vi "LVClass_WavefrontCorrector Check User Preferences.vi"(0 "WavefrontCorrector in":refnum<class "WavefrontCorrector.lvclass">, 5 "Mirror preferences":T1, 11 "error in (no error)":errorcluster) -> (4 "WavefrontCorrector out":refnum<class "WavefrontCorrector.lvclass">, 15 "error out":errorcluster)   [LabVIEW 2020, in "WavefrontCorrector.lvclass"]
doc: "Assert requested preferences fulfill specifications constraints.\n\n--------------------------------------------------------------------------------\n\n<B>correctorIn </B> : WavefrontCorrector object.\n<B>correctorOut </B> : WavefrontCorrector object.\n<B>sleep_after_movement </B> : WavefrontCorrector preferences : Time to stabilization (ms).\n<B>min </B> : WavefrontCorrector preferences : lowest command value.\n<B>max </B> : WavefrontCorrector preferences : highest command value.\n<B>validity </B> : WavefrontCorrector preferences : status.\n<B>fixed_values </B> : WavefrontCorrector preferences : fixed positions.\n<B>ErrorIn </B> : Error\n<B>ErrorOut </B> : Error\n\n--------------------------------------------------------------------------------"
uses:
  WavefrontCorrector.lvclass
  Wavefront Corrector states.ctl
  Wavefront Corrector states - ONE.ctl
  WavefrontCorrector.lvclass/WavefrontCorrector.ctl
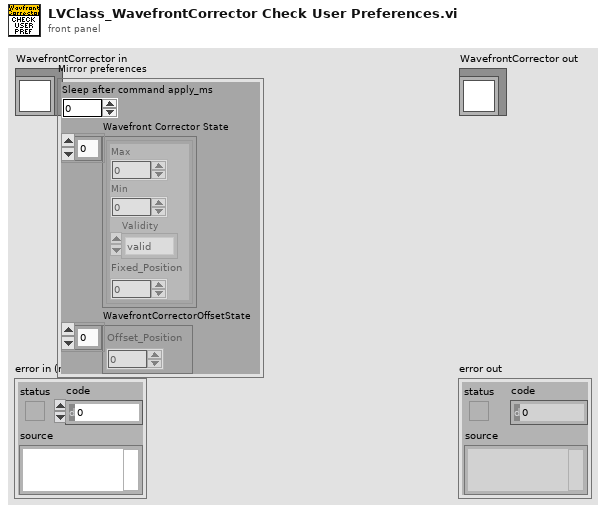
[diagram p1: front panel]
types:
  T1 = typedef "Wavefront Corrector states.ctl" = cluster{"Sleep after command apply_ms":i32, "Wavefront Corrector State":T2[], "WavefrontCorrectorOffsetState":sgl[]}
  T2 = typedef "Wavefront Corrector states - ONE.ctl" = cluster{"Max":sgl, "Min":sgl, "Validity":enum16{"valid", "fixed", "invalid"}, "Fixed_Position":sgl}
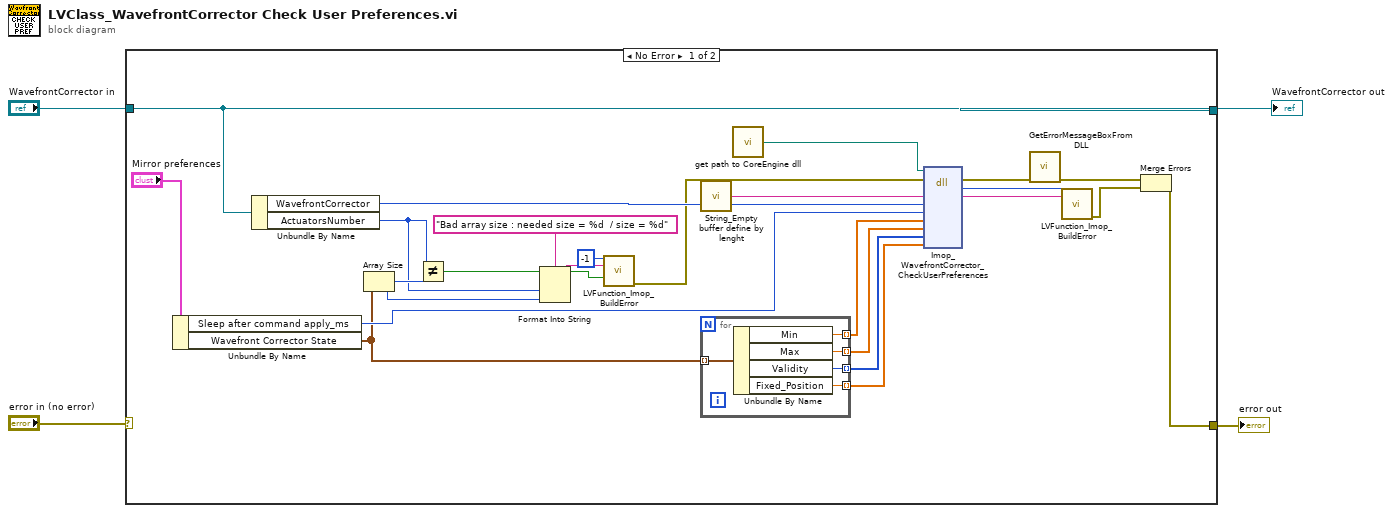
[diagram p0: block diagram]
diagram:
  n1 = case shown="No Error" "error in (no error)" {
    selector: "error in (no error)" -> [_ w35]
    tunnel: [w26 w35] -> w1
    tunnel: [w25 w34] -> w2
    tunnel: "WavefrontCorrector in" -> [w25 w34]
    frame No Error {
      n2 = Unbundle By Name("Mirror preferences") -> ("Sleep after command apply_ms"=w19:i32, "Wavefront Corrector State"=w18:T2[])
      n3 = Unbundle By Name(w25) -> ("WavefrontCorrector"=w24:i32, "ActuatorsNumber"=w14:i32)
      n4 = Array Size(array=w18) -> (size(s)=w15:i32)
      n5 = Not Equal?(x=w14, y=w15) -> (x != y?=w9:bool)
      n6 = Format Into String(format string="Bad array size : needed size = %d  / size = %d" ("String to Prepend to source (\"\")"), w14, w15) -> (resulting string=w16:string)  [unwired: 2 in, 1 out]
      n7 = call "LVFunction_Imop_BuildError.vi"("code"=-1, "String to Prepend to source (\"\")"=w16, "Activate error? (true)"=w9) -> ("error out"=w7:errorcluster)  [unwired: 12 in]
      n8 = call "String_Empty buffer define by lenght.vi"() -> ("Empty buffer"=w12:string)  [unwired: 1 in]
      n9 = for {
        tunnel: w18 -> [w33] mode=indexing
        tunnel: [w32] -> w6 mode=indexing
        tunnel: [w31] -> w5 mode=indexing
        tunnel: [w30] -> w11 mode=indexing
        tunnel: [w29] -> w10 mode=indexing
        n10 = Unbundle By Name(w33) -> ("Min"=w32:sgl, "Max"=w31:sgl, "Validity"=w30:enum16{"valid", "fixed", "invalid"}, "Fixed_Position"=w29:sgl)
      }
      n11 = call "get path to CoreEngine dll.vi"() -> ("path to c_interface_vc100.dll"=w13:path)  [unwired: 12 in, 3 out]
      n12 = dll-call lib="D:/SOFTware/HASO_v3/SVN_trunk/ImOpCoreEngine4_LV2011/DLLs/c_interface_vc100.dll" fn="Imop_WavefrontCorrector_CheckUserPreferences"(path in=w13, error in=w7, "message"=w12, "WavefrontCorrection"=w24, "sleep_after_movement"=w19, "min"=w6, "max"=w5, "validity"=w11, "fixed_value"=w10) -> (error out=w23:errorcluster, "return type"=w22:i32, "message"=w21:string)  [unwired: 7 in, 1 out]
      n13 = call "GetErrorMessageBoxFromDLL.vi"("error IN"=w23) -> ("error OUT"=w28:errorcluster)  [unwired: 10 in]
      n14 = call "LVFunction_Imop_BuildError.vi"("code"=w22, "String to Prepend to source (\"\")"=w21) -> ("error out"=w27:errorcluster)  [unwired: 13 in]
      n15 = Merge Errors(w28, w27) -> (w26:errorcluster)
    }
    frame Error {
    }
  }
  "error out" <- w1
  "WavefrontCorrector out" <- w2
